vi "load.vi"(8 "error in (no error)":errorcluster) -> (0 "error out":errorcluster, 3 "preregistraion_data":T1={"Hardware version"="HW01.02", "Order number"="31735", "Model number"="800688", "Starting serial number"=0, "Starting MAC address"="", "Ending MAC address"="", "TKE_LOT_SIZE"=0} {"Starting serial number" format="%#_11g"})   [LabVIEW 2018]
uses:
  controls/preregistration_data.ctl
  <vilib>/Utility/sysdir.llb/System Directory Type.ctl
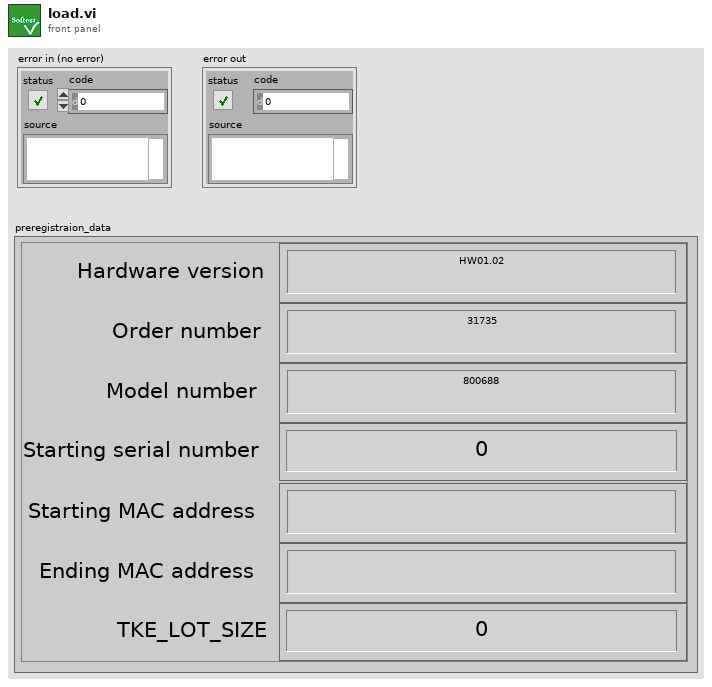
[diagram p1: front panel]
types:
  T1 = typedef "preregistration_data.ctl" = cluster{"Hardware version":string, "Order number":string, "Model number":string, "Starting serial number":i32, "Starting MAC address":string, "Ending MAC address":string, "TKE_LOT_SIZE":i32}
  T2 = typedef "System Directory Type.ctl" = i32
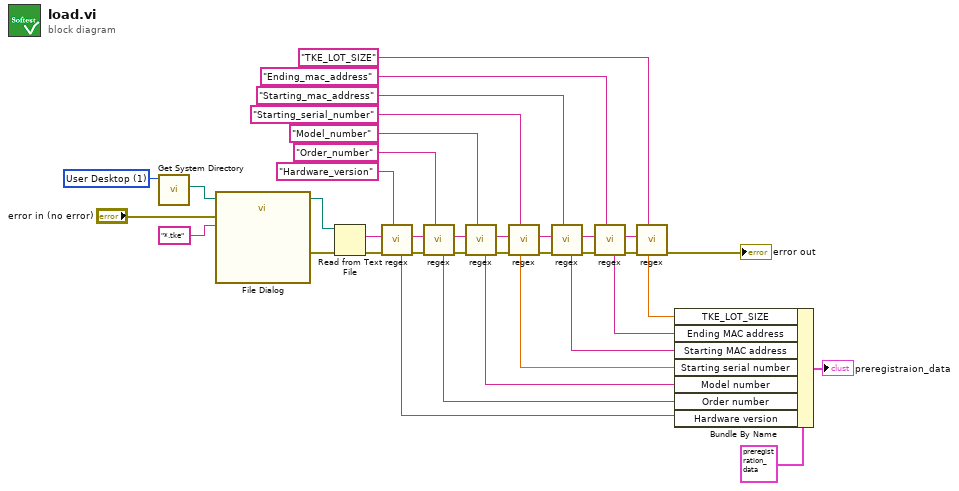
[diagram p0: block diagram]
diagram:
  w35 = T2 1 items=["User Home"=0, "User Desktop"=1, "User Documents"=2, "User Application Data"=3, "User Preferences"=4, "User Temporary"=5, "Public Documents"=6, "Public Application Data"=7, "Public Preferences"=8, "Public Cache"=13, "System Core Libraries"=9, "System Installed Libraries"=10, "Application Files"=11, "Boot Volume Root"=12] ("system directory type")
  n1 = call <vilib>:"Get System Directory.vi"("system directory type"=w35) -> ("system directory"=w36:path)  [unwired: 10 in]
  n2 = call "File Dialog"("start path"=w36, "error in"="error in (no error)", "pattern (all files)"="*.tke") -> ("selected path"=w32:path, "error out"=w34:errorcluster)  [unwired: 9 in, 2 out]
  n3 = Read from Text File(file (use dialog)=w32, error in=w34) -> (text=w29:string, error out=w31:errorcluster)  [unwired: 2 in, 2 out]
  n4 = call "regex.vi"("property_name"="Hardware_version" ("regular expression"), "error_in"=w31, "preregistration_data_content_in"=w29) -> ("error_out"=w28:errorcluster, "preregistration_data_content_out"=w26:string, "property_value"=w8:string)  [unwired: 5 in, 1 out]
  n5 = call "regex.vi"("property_name"="Order_number" ("regular expression"), "error_in"=w28, "preregistration_data_content_in"=w26) -> ("error_out"=w27:errorcluster, "preregistration_data_content_out"=w25:string, "property_value"=w7:string)  [unwired: 5 in, 1 out]
  n6 = call "regex.vi"("property_name"="Model_number" ("regular expression"), "error_in"=w27, "preregistration_data_content_in"=w25) -> ("error_out"=w24:errorcluster, "preregistration_data_content_out"=w23:string, "property_value"=w6:string)  [unwired: 5 in, 1 out]
  n7 = call "regex.vi"("property_name"="Starting_serial_number" ("regular expression"), "error_in"=w24, "preregistration_data_content_in"=w23) -> ("error_out"=w22:errorcluster, "preregistration_data_content_out"=w21:string, "property_value_num"=w2:dbl)  [unwired: 5 in, 1 out]
  n8 = call "regex.vi"("property_name"="Starting_mac_address" ("regular expression"), "error_in"=w22, "preregistration_data_content_in"=w21) -> ("error_out"=w20:errorcluster, "preregistration_data_content_out"=w19:string, "property_value"=w5:string)  [unwired: 5 in, 1 out]
  n9 = call "regex.vi"("property_name"="Ending_mac_address" ("regular expression"), "error_in"=w20, "preregistration_data_content_in"=w19) -> ("error_out"=w18:errorcluster, "preregistration_data_content_out"=w17:string, "property_value"=w4:string)  [unwired: 5 in, 1 out]
  n10 = call "regex.vi"("property_name"="TKE_LOT_SIZE" ("regular expression"), "error_in"=w18, "preregistration_data_content_in"=w17) -> ("error_out"=→"error out":errorcluster, "property_value_num"=w1:dbl)  [unwired: 5 in, 2 out]
  n11 = Bundle By Name(cluster=T1 {"Hardware version"="HW01.02", "Order number"="31735", "Model number"="800688", "Starting serial number"=0, "Starting MAC address"="", "Ending MAC address"="", "TKE_LOT_SIZE"=0} ("preregistration_data"), "TKE_LOT_SIZE"=w1, "Ending MAC address"=w4, "Starting MAC address"=w5, "Starting serial number"=w2, "Model number"=w6, "Order number"=w7, "Hardware version"=w8) -> (→"preregistraion_data":T1)
